vi "RVC Denavit-Hartenberg Link.vi"() -> ()   [LabVIEW 2013]
uses:
  <vilib>/robotics/Kinematics/Link/Joint Type.ctl
  <vilib>/robotics/Kinematics/DH Kinematic Parameters.ctl
  <vilib>/robotics/Kinematics/Analytical/Initialize Generic Serial Arm.vi
  <vilib>/robotics/Kinematics/Analytical/NI_Robotics_AnalyticKinematics.lvlib
  <vilib>/robotics/Kinematics/Robot/NI_Robotics_Serial Robot Arm.lvclass
  <vilib>/robotics/Kinematics/Link/NI_Robotics_Link.lvclass
  <vilib>/robotics/Kinematics/NI_Kinematics.lvlib
panel:
  out "L.A (0) with offset":picture
  out "joint type":T1
  out "a":dbl
  out "L.A (.0.5)":picture
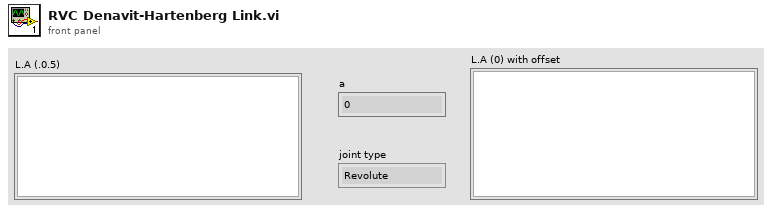
[diagram p1: front panel]
types:
  T1 = typedef "NI_Robotics_Link.lvclass/Joint Type.ctl" = enum16{"Revolute", "Prismatic"}
  T2 = typedef "DH Kinematic Parameters.ctl" = cluster{"twist angle":dbl, "length":dbl, "rotation angle":dbl, "offset distance":dbl, "joint type":T1, "joint coordinate offset":dbl}
  T3 = typedef "NI_Matrix.lvlib/RealMatrix.ctl" = dbl[][]
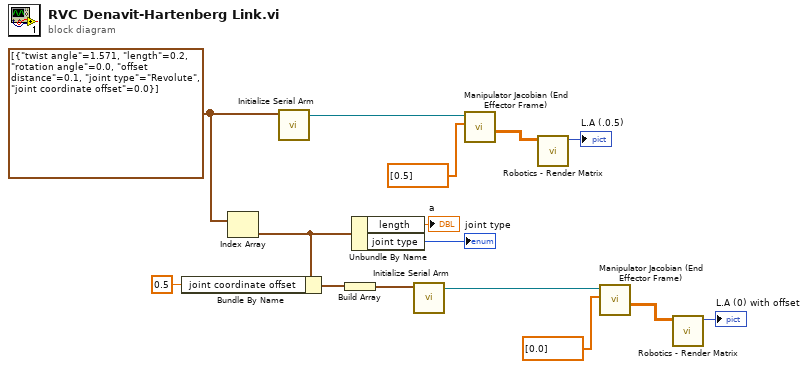
[diagram p0: block diagram]
diagram:
  w11 = T2[] [{"twist angle"=1.571, "length"=0.2, "rotation angle"=0.0, "offset distance"=0.1, "joint type"=enum."Revolute", "joint coordinate offset"=0.0}] ("kinematic parameters")
  n1 = Index Array(array=w11) -> (element=w4:T2)  [unwired: 1 in]
  n2 = Bundle By Name(cluster=w4, "joint coordinate offset"=0.5) -> (w3:T2)
  n3 = call-poly <vilib>:"Initialize Serial Arm.vi"("kinematic parameters"=w11) -> ("serial arm out"=w12:refnum<class "NI_Robotics_Serial Robot Arm.lvclass">)  [unwired: 9 in, 1 out]
  n4 = Build Array(w3) -> (w2:T2[])
  n5 = Unbundle By Name(w4) -> ("length"=→"a":dbl, "joint type"=→"joint type":T1)
  n6 = call-poly <vilib>:"Initialize Serial Arm.vi"("kinematic parameters"=w2) -> ("serial arm out"=w8:refnum<class "NI_Robotics_Serial Robot Arm.lvclass">)  [unwired: 9 in, 1 out]
  n7 = call <vilib>:"Manipulator Jacobian (End Effector Frame).vi"("joint positions"=dbl[] [0.5], "serial arm in"=w12) -> ("forward kinematics"=w13:T3)  [unwired: 6 in, 3 out]
  n8 = call "Robotics - Render Matrix.vi"("A"=w13) -> ("picture out"=→"L.A (.0.5)":picture)  [unwired: 10 in]
  n9 = call <vilib>:"Manipulator Jacobian (End Effector Frame).vi"("joint positions"=dbl[] [0.0], "serial arm in"=w8) -> ("forward kinematics"=w7:T3)  [unwired: 6 in, 3 out]
  n10 = call "Robotics - Render Matrix.vi"("A"=w7) -> ("picture out"=→"L.A (0) with offset":picture)  [unwired: 10 in]
